vi "Configure Control.vi"(8 "error in (no error)":errorcluster, 10 "control in":refnum<vi>, 11 "Base in":refnum<class "Base.lvclass">) -> (0 "error out":errorcluster, 2 "control out":refnum<vi>, 3 "Base out":refnum<class "Base.lvclass">)   [LabVIEW 2020, in "PV Access.lvlib" / "PV Data.lvlib" / "Base.lvclass"]
doc: "Set the description of <B>control</B> from the value's metadata."
uses:
  Base.lvclass
  Base.lvclass/Base.ctl
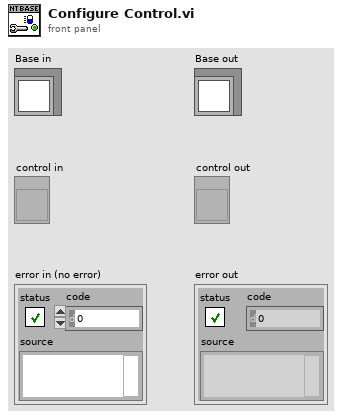
[diagram p1: front panel]
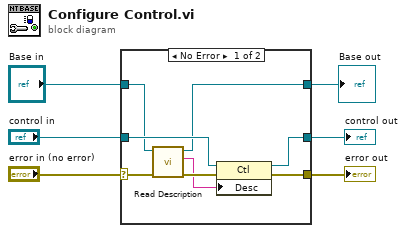
[diagram p0: block diagram]
diagram:
  n1 = case shown="No Error" "error in (no error)" {
    selector: "error in (no error)" -> [w9 w17]
    tunnel: [w13 w17] -> w5
    tunnel: [w11 w16] -> w3
    tunnel: "Base in" -> [w12 w16]
    tunnel: "control in" -> [w14 w15]
    tunnel: [w10 w15] -> w1
    frame No Error {
      n2 = call-dynamic "Read Description.vi"("error in (no error)"=w9, "Base Interface in"=w12) -> ("error out"=w8:errorcluster, "description"=w7:string, "Base Interface out"=w11:refnum<class "Base.lvclass">)  [unwired: 7 in]
      n3 = property class="Ctl"(reference=w14, error in=w8, "Desc"=w7) -> (reference out=w10:refnum<vi>, error out=w13:errorcluster)
    }
    frame Error {
    }
  }
  "error out" <- w5
  "Base out" <- w3
  "control out" <- w1
